vi "Set Transfer Groups.vi"(10 "Transfer Groups":refnum<class "Transfer Group.lvclass">[](array[class]), 11 "Transceiver Thread in":refnum<class "Transceiver Thread.lvclass">) -> (3 "Transceiver Thread out":refnum<class "Transceiver Thread.lvclass">)   [LabVIEW 2017, in "Data Sharing Framework Core.lvlib" / "Data Sharing Framework Engine.lvlib" / "Transceiver Thread.lvclass"]
uses:
  Transceiver Thread.lvclass
  Transfer Group/Transfer Group.lvclass
  Transceiver Thread.lvclass/Transceiver Thread.ctl
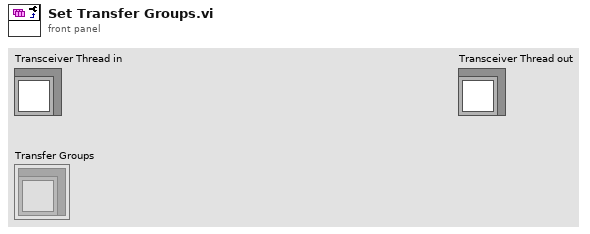
[diagram p1: front panel]
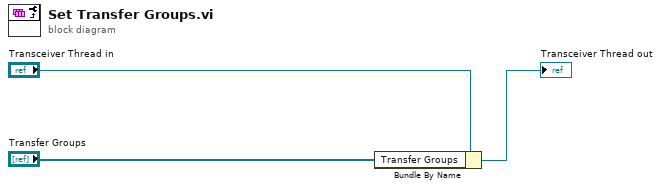
[diagram p0: block diagram]
diagram:
  n1 = Bundle By Name(cluster="Transceiver Thread in", "Transfer Groups"="Transfer Groups") -> (→"Transceiver Thread out":refnum<class "Transceiver Thread.lvclass">)
